vi "ErrorToLogFormat.vi"(8 "error in (no error)":errorcluster, 10 "ReportedError":errorcluster, 11 "Count":i32) -> (0 "error out":errorcluster, 3 "Log format":string)   [LabVIEW 2018, in "ErrorLogFile.lvclass"]
uses:
  ErrorLogFile.lvclass
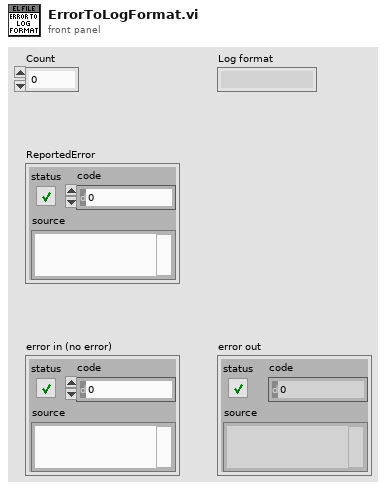
[diagram p1: front panel]
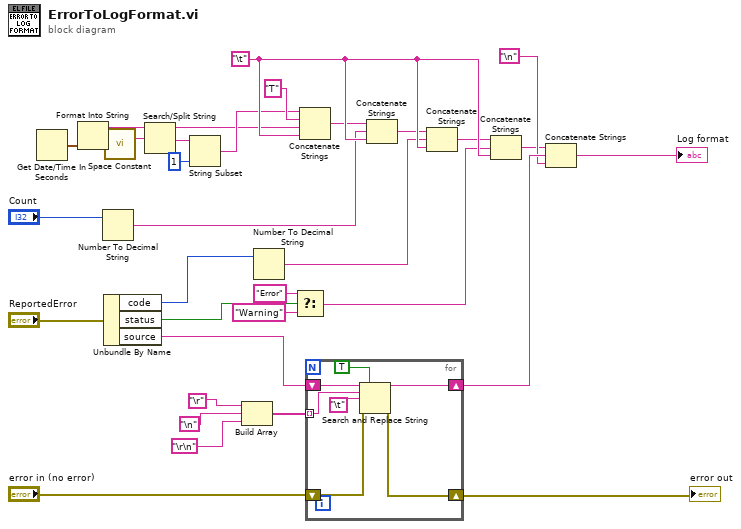
[diagram p0: block diagram]
diagram:
  w21 = "\t"
  n1 = Get Date/Time In Seconds() -> (seconds since 1Jan1904=w2:timestamp)
  n2 = Format Into String(w2) -> (resulting string=w3:string)  [unwired: 3 in, 1 out]
  n3 = Number To Decimal String(number="Count") -> (decimal integer string=w11:string)  [unwired: 1 in]
  n4 = Unbundle By Name("ReportedError") -> ("code"=w14:i32, "status"=w18:bool, "source"=w30:string)
  n5 = call <vilib>:"Space Constant.vi"() -> ("String"=w4:string)
  n6 = Search/Split String(string=w3, search string/char (-)=w4) -> (substring before match=w5:string, match + rest of string=w6:string)  [unwired: 1 in, 1 out]
  n7 = String Subset(string=w6, offset (0)=1) -> (substring=w8:string)  [unwired: 1 in]
  n8 = Build Array("\r", "\n", "\r\n") -> (w27:string[])
  n9 = Number To Decimal String(number=w14) -> (decimal integer string=w15:string)  [unwired: 1 in]
  n10 = Select(t="Error", s=w18, f="Warning") -> (s? t:f=w20:string)
  n11 = Concatenate Strings(w8, "T" ("string"), w5, w21) -> (w10:string)
  n12 = for {
    tunnel: w27 -> [w36] mode=indexing
    shift-right: [w37] -> w31
    shift-left: w30 -> [w39]
    shift-right: [w33] -> w29
    shift-left: "error in (no error)" -> [w34]
    n13 = Search and Replace String(replace all?=TRUE ("replace all? (F)"), input string=w39, search string=w36, replace string="\t", error in=w34) -> (result string=w37:string, error out=w33:errorcluster)  [unwired: 3 in, 2 out]
  }
  "error out" <- w29
  n14 = Concatenate Strings(w10, w11, w21) -> (w12:string)
  n15 = Concatenate Strings(w12, w15, w21) -> (w19:string)
  n16 = Concatenate Strings(w19, w20, w21) -> (w22:string)
  n17 = Concatenate Strings(w22, w31, "\n") -> (→"Log format":string)
